vi "Configure Channel (Voltage).vi"(4 "Power Line Cycles (0)":i32, 5 "Current Limit (1.0 uA)":dbl=1e-06, 6 "Triggered Level (1.0 V)":dbl=1.0, 7 "Voltage Range (0: 2 Volts)":u16(ring) items=["2 Volts", "20 Volts"], 8 "error in (no error)":errorcluster, 9 "Output Level (1.0 V)":dbl=1.0, 10 "Channel (1: Channel 1)":u16(ring)=1 items=["Channel 1"=1, "Channel 2"=2, "Channel 3"=3], 11 "VISA resource name":refnum<visa-resource-name>) -> (0 "error out":errorcluster, 3 "VISA resource name out":refnum<visa-resource-name>)   [LabVIEW 2010, in "Agilent U2722.lvlib"]
doc: "Configures the channel to output in source voltage mode."
uses:
  Agilent U2722.lvlib
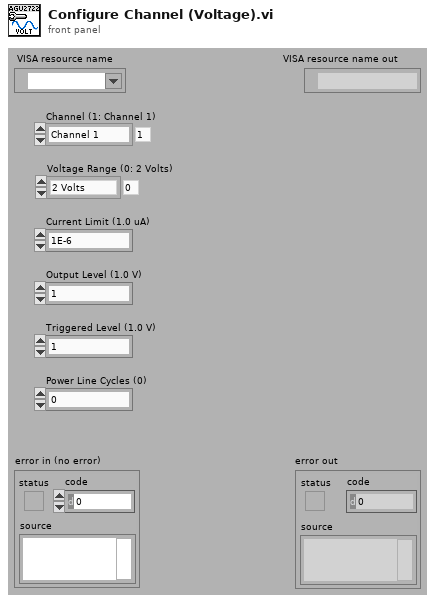
[diagram p1: front panel]
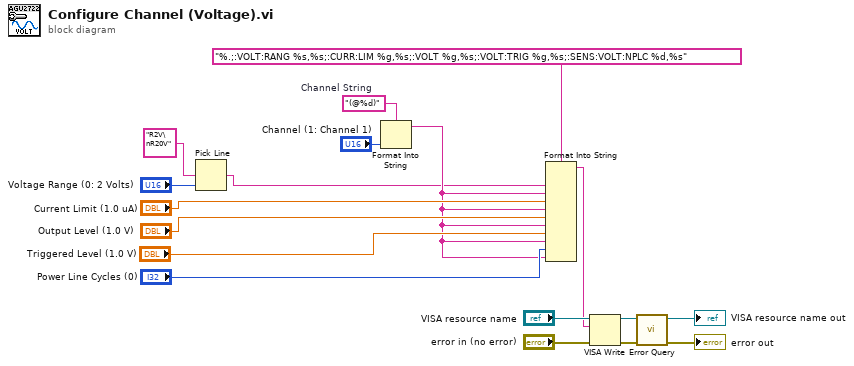
[diagram p0: block diagram]
diagram:
  w11 = "(@%d)"  # Channel String
  n1 = Pick Line(multi-line string="R2V\nR20V", line index="Voltage Range (0: 2 Volts)") -> (output string=w1:string)  [unwired: 1 in]
  n2 = Format Into String(format string=w11, "Channel (1: Channel 1)") -> (resulting string=w5:string)  [unwired: 2 in, 1 out]
  n3 = Format Into String(format string="%.;:VOLT:RANG %s,%s;:CURR:LIM %g,%s;:VOLT %g,%s;:VOLT:TRIG %g,%s;:SENS:VOLT:NPLC %d,%s", w1, w5, "Current Limit (1.0 uA)", w5, "Output Level (1.0 V)", w5, "Triggered Level (1.0 V)", w5, "Power Line Cycles (0)", w5) -> (resulting string=w4:string)  [unwired: 2 in, 1 out]
  n4 = VISA Write(VISA resource name="VISA resource name", write buffer=w4, error in (no error)="error in (no error)") -> (VISA resource name out=w14:refnum<visa-resource-name>, error out=w13:errorcluster)  [unwired: 1 out]
  n5 = call "Error Query.vi"("error in (no error)"=w13, "VISA resource name"=w14) -> ("error out"=→"error out":errorcluster, "VISA resource name out"=→"VISA resource name out":refnum<visa-resource-name>)  [unwired: 6 in, 2 out]
